vi "DSF.Engine.Debug Flags.Get FIFO Flags.vi"(11 "Debug Flags in":refnum<class "DSF.Engine.Debug Flags.lvclass">) -> (2 "FIFO":refnum<class "DSF.Engine.Debug Flags.FIFO.lvclass">, 3 "Debug Flags out":refnum<class "DSF.Engine.Debug Flags.lvclass">)   [LabVIEW 2017, in "DSF.Engine.lvlib" / "DSF.Engine.Debug Flags.lvclass"]
uses:
  DSF.Engine.Debug Flags.lvclass
  DSF.Engine.Debug Flags.FIFO.lvclass
  DSF.Engine.Debug Flags.lvclass/DSF.Engine.Debug Flags.ctl
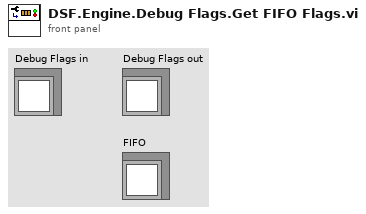
[diagram p1: front panel]
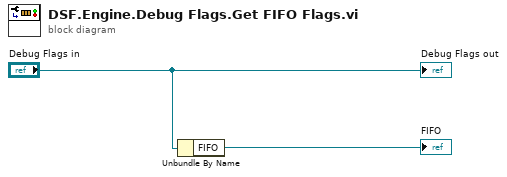
[diagram p0: block diagram]
diagram:
  n1 = Unbundle By Name("Debug Flags in") -> ("FIFO"=→"FIFO":refnum<class "DSF.Engine.Debug Flags.FIFO.lvclass">)
  "Debug Flags out" <- "Debug Flags in"
